vi "UART 8N1 Cleanup Acquisition Buffer.vi"(8 "Active Dut":T1, 10 "Error In":errorcluster, 11 "FPGA VI Reference In":refnum<k20>) -> (1 "Elements Remaining":u32, 2 "Error Out":errorcluster, 3 "FPGA VI Reference Out":refnum<k20>)   [LabVIEW 2018]
uses:
  Resources_Test/UART/ControlTestSlot.ctl
  <vilib>/Utility/error.llb/Error Cluster From Error Code.vi
  <vilib>/rvi/errors/niLvFpgaAdjustHostInterfaceError.vi
  <vilib>/rvi/interface/nirviMethod/nirviMethod.xnode
  Program Files (x86)/National Instruments/LabVIEW 2018/instr.lib/niVST/FPGA/Templates/FPGA Bitfiles/niVSTFPGA_UART.lvbitx
  <vilib>/rvi/errors/niLvFpgaMergeErrorWithErrorCode.vi
  <vilib>/FPGAPlugInAG/PXIe-5840/niLvFpga_ReadFifo_PXIe-5840.vi
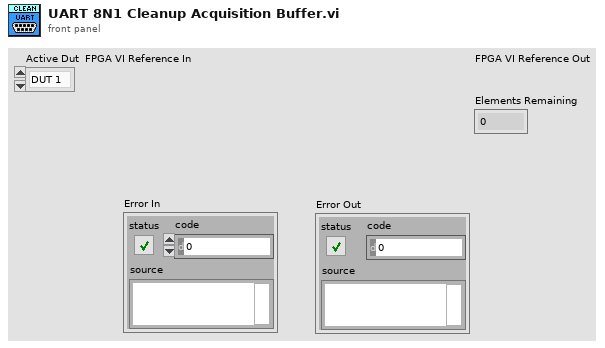
[diagram p1: front panel]
types:
  T1 = typedef "ControlTestSlot.ctl" = enum16{"DUT 1", "DUT 2"}
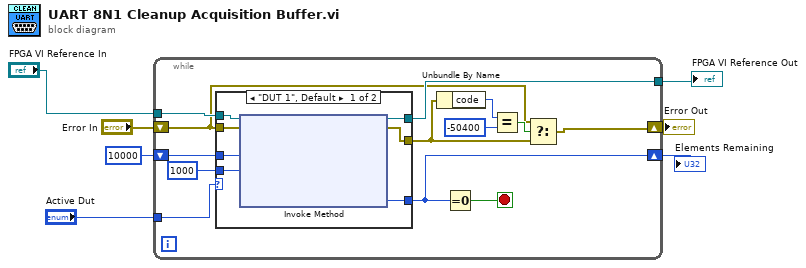
[diagram p0: block diagram]
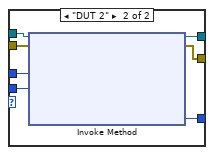
[diagram p2: hidden frame]
diagram:
  n1 = while {
    shift-right: [w9] -> w6
    shift-left: "Error In" -> [w11]
    tunnel: "FPGA VI Reference In" -> [w20]
    tunnel: [w19] -> w3
    shift-right: [w16] -> w1
    shift-left: u32 10000 ("Response Size (char)") -> [w17]
    tunnel: "Active Dut" -> [w8]
    stop <- w18 stop-if-true
    n2 = case shown="\"DUT 1\", Default" w8 {
      tunnel: w11 -> [w24 w34]
      tunnel: w20 -> [w25 w33]
      tunnel: [w27 w32] -> w10
      tunnel: [w26 w31] -> w19
      tunnel: [w23 w30] -> w16
      tunnel: w17 -> [w22 w29]
      tunnel: 1000 ("Response Timeout (ms)") -> [w21 w28]
      frame "DUT 1", Default {
        n3 = xnode "Invoke Method"("FPGA VI Reference In"=w25, "error in"=w24, "Number of Elements"=w22, "Timeout (ms)"=w21) -> ("FPGA VI Reference Out"=w26:refnum<k20>, "error out"=w27:errorcluster, "Elements Remaining"=w23:u32)  [unwired: 1 out]
      }
      frame "DUT 2" {
        n4 = xnode "Invoke Method"("FPGA VI Reference In"=w33, "error in"=w34, "Number of Elements"=w29, "Timeout (ms)"=w28) -> ("FPGA VI Reference Out"=w31:refnum<k20>, "error out"=w32:errorcluster, "Elements Remaining"=w30:u32)  [unwired: 1 out]
      }
    }
    n5 = Unbundle By Name(w10) -> ("code"=w13:i32)
    n6 = Equal To 0?(x=w16) -> (x = 0?=w18:bool)
    n7 = Equal?(x=w13, y=-50400) -> (x = y?=w14:bool)
    n8 = Select(t=w11, s=w14, f=w10) -> (s? t:f=w9:errorcluster)
  }
  "Error Out" <- w6
  "FPGA VI Reference Out" <- w3
  "Elements Remaining" <- w1
